vi "Get ctrl Primary Axis.vi"(3 "Axis Actions":T1) -> (0 "Axis Primary":dbl)   [LabVIEW 2014]
uses:
  Axis Actions.ctl
  SRE Enum.ctl
  Support Code/Robot Global Data.vi
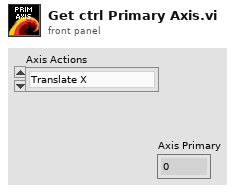
[diagram p1: front panel]
types:
  T1 = typedef "Axis Actions.ctl" = enum16{"Translate X", "Translate Y", "Rotate"}
  T2 = enum16{"X left ", "Y left", "Z left", "X right", "Y right", "Z right"}[]
  T3 = typedef "SRE Enum.ctl" = enum16{"Start", "Run", "End"}
  T4 = enum16{"X left ", "Y left", "Z left", "X right", "Y right", "Z right"}
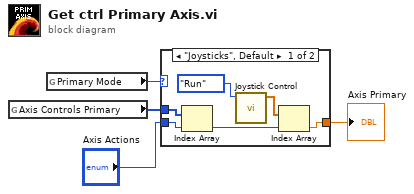
[diagram p0: block diagram]
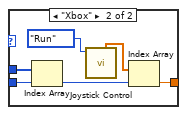
[diagram p2: hidden frame]
diagram:
  n1 = global read "Robot Global Data.vi" "Axis Controls Primary"() -> (w3:T2)
  n2 = global read "Robot Global Data.vi" "Primary Mode"() -> (w4:enum16{"Joysticks", "Xbox"})
  n3 = case shown="\"Joysticks\", Default" w4 {
    tunnel: w3 -> [w6 w14]
    tunnel: "Axis Actions" -> [w5 w13]
    tunnel: [w7 w11] -> w1
    frame "Joysticks", Default {
      n4 = Index Array(array=w6, index=w5) -> (element=w10:T4)
      n5 = call "Joystick Control.vi"("Enum"=SRE_Enum."Run") -> ("Axis Output PJ"=w8:dbl[])  [unwired: 3 in, 5 out]
      n6 = Index Array(array=w8, index=w10) -> (element=w7:dbl)
    }
    frame "Xbox" {
      n7 = Index Array(array=w14, index=w13) -> (element=w16:T4)
      n8 = call "Joystick Control.vi"("Enum"=SRE_Enum."Run") -> ("Axis Output PX"=w12:dbl[])  [unwired: 3 in, 5 out]
      n9 = Index Array(array=w12, index=w16) -> (element=w11:dbl)
    }
  }
  "Axis Primary" <- w1
